vi "In Range.vi"(9 "Tolerance":dbl, 10 "Encoder Height":dbl, 11 "Height":dbl) -> (3 "In Range":bool)   [LabVIEW 2017]
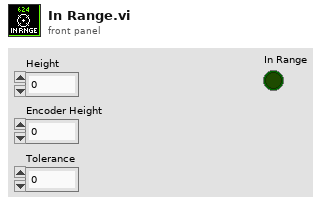
[diagram p1: front panel]
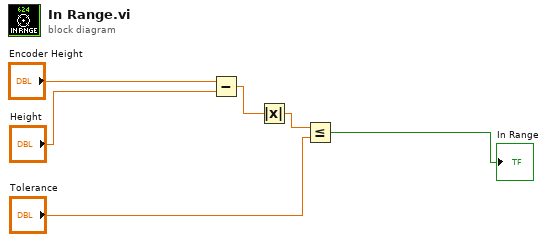
[diagram p0: block diagram]
diagram:
  n1 = Subtract(x="Encoder Height", y="Height") -> (x-y=w4:dbl)
  n2 = Absolute Value(x=w4) -> (abs(x)=w3:dbl)
  n3 = Less Or Equal?(x=w3, y="Tolerance") -> (x <= y?=→"In Range":bool)
